vi "Scan Timestamp.vi"(8 "error in (no error)":errorcluster, 11 "String":string) -> (0 "error out":errorcluster, 3 "Timestamp":timestamp)   [LabVIEW 2011, in "JSON Scalar.lvclass"]
uses:
  JSON Scalar.lvclass
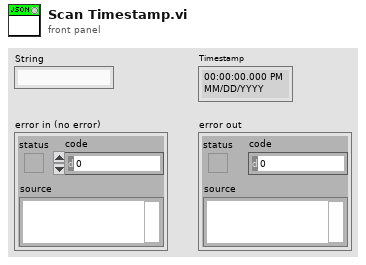
[diagram p1: front panel]
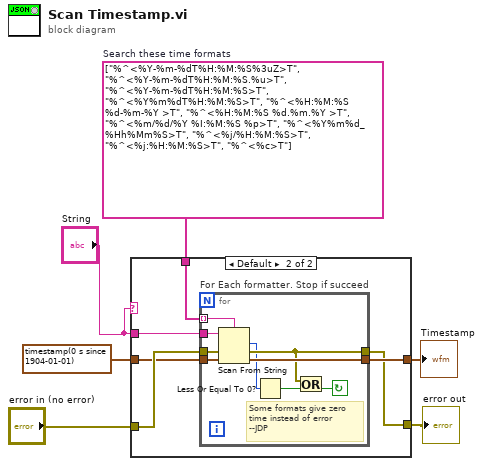
[diagram p0: block diagram]
diagram:
  w6 = string[] ["%^<%Y-%m-%dT%H:%M:%S%3uZ>T", "%^<%Y-%m-%dT%H:%M:%S.%u>T", "%^<%Y-%m-%dT%H:%M:%S>T", "%^<%Y%m%dT%H:%M:%S>T", "%^<%H:%M:%S %d-%m-%Y >T", "%^<%H:%M:%S %d.%m.%Y >T", "%^<%m/%d/%Y %I:%M:%S %p>T", "%^<%Y%m%d_%Hh%Mm%S>T", "%^<%j/%H:%M:%S>T", "%^<%j:%H:%M:%S>T", "%^<%c>T"]  # Search these time formats
  n1 = case shown="Default" "String" {
    tunnel: [w7 w14] -> w1
    tunnel: "error in (no error)" -> [w8 w13]
    tunnel: [w8 w12] -> w3
    tunnel: timestamp(0 s since 1904-01-01) ("default value 1") -> [w7 w11]
    tunnel: "String" -> [_ w10]
    tunnel: w6 -> [_ w9]
    frame "null" {
    }
    frame Default {
      n2 = for "For Each formatter. Stop if succeed" {
        tunnel: [w23] -> w14
        tunnel: w13 -> [w22]
        tunnel: [w16] -> w12
        tunnel: w11 -> [w21]
        tunnel: w10 -> [w20]
        tunnel: w9 -> [w19] mode=indexing
        stop <- w17 continue-if-true
        # "Some formats give zero\ntime instead of error\n--JDP"
        n3 = Scan From String(format string=w19, input string=w20, error in=w22, default 1=w21) -> (offset past scan=w15:u32, error out=w16:errorcluster, output 1=w23:timestamp)  [unwired: 1 in, 1 out]
        n4 = Less Or Equal To 0?(x=w15) -> (x <= 0?=w18:bool)
        n5 = Or(x=w16, y=w18) -> (x .or. y?=w17:bool)
      }
    }
  }
  "error out" <- w3
  "Timestamp" <- w1
